vi "GetConnections.vi"(5 "Terminals":refnum<class "Terminal.lvclass">[](array[class]), 9 "Wire in":refnum<class "Wire.lvclass">) -> (3 "Wire out":refnum<class "Wire.lvclass">)   [LabVIEW 2014, in "Raspberry Pi Compatible Compiler for LabVIEW.lvlib" / "Wire.lvclass"]
uses:
  Wire.lvclass
  Terminal/Terminal.lvclass
  ConnectionsTD.ctl
  Wire.lvclass/Wire.ctl
  Raspberry Pi Compatible Compiler for LabVIEW.lvlib
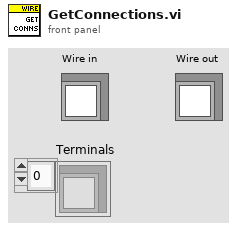
[diagram p1: front panel]
types:
  T1 = typedef "Raspberry Pi Compatible Compiler for LabVIEW.lvlib/ConnectionsTD.ctl" = cluster{"source":refnum<class "Terminal.lvclass">, "sink":refnum<class "Terminal.lvclass">}
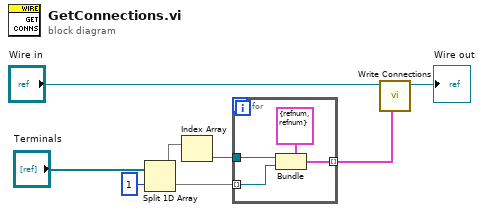
[diagram p0: block diagram]
diagram:
  n1 = Split 1D Array(array="Terminals", index=1) -> (first subarray=w7:refnum<class "Terminal.lvclass">[], second subarray=w5:refnum<class "Terminal.lvclass">[])
  n2 = Index Array(array=w7) -> (element=w6:refnum<class "Terminal.lvclass">)  [unwired: 1 in]
  n3 = for {
    tunnel: w6 -> [w10]
    tunnel: w5 -> [w9] mode=indexing
    tunnel: [w11] -> w4 mode=indexing
    n4 = Bundle(cluster=T1 {"source"=refnum, "sink"=refnum}, "source"=w10, "sink"=w9) -> (w11:T1)
  }
  n5 = call "Write Connections.vi"("Connections"=w4, "Wire in"="Wire in") -> ("Wire out"=→"Wire out":refnum<class "Wire.lvclass">)  [unwired: 7 in]
